vi "testIsTelQueueFull.vi"(8 "error in (no error)":errorcluster) -> (0 "error out":errorcluster)   [LabVIEW 2018]
doc: "Test the isTelQueueFull.vi."
uses:
  src/TcpServer/TcpServer.lvclass
  src/TcpServerTel/typedef/enqueueOptionsTypeDef.ctl
  src/TcpServerTel/typedef/queueOptionsTypeDef.ctl
  src/TcpServer/TcpServer.lvclass/TcpServer.ctl
  src/TcpServerTel/typedef/telTypeDef.ctl
  src/TcpServerBase/TcpServerBase.lvclass/TcpServerBase.ctl
  src/TcpServerTel/TcpServerTel.lvclass
  home/pcortes/github/ts_labview_tcp_json/src/TcpServerBase/TcpServerBase.lvclass
  <vilib>/addons/_JKI Toolkits/Caraya/classes/Assert/Assert False.vi
  <vilib>/addons/_JKI Toolkits/Caraya/classes/Assert/Assert True.vi
  <vilib>/addons/_JKI Toolkits/Caraya/classes/Test/Test.lvclass
  <vilib>/addons/_JKI Toolkits/Caraya/classes/Assert/Assert.lvclass
  src/TcpServerBase/TcpServerBase.lvclass
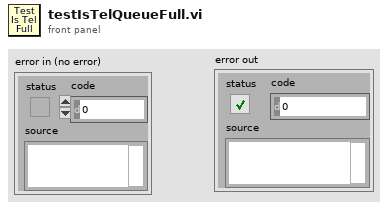
[diagram p1: front panel]
types:
  T1 = typedef "TcpServerTel.lvclass/enqueueOptionsTypeDef.ctl" = enum16{"lossy enqueue", "normal enqueue"}
  T2 = typedef "TcpServerTel.lvclass/queueOptionsTypeDef.ctl" = cluster{"EnqueueOptions":T1, "Timeout":i32}
  T3 = cluster{"cmdServerPort":u16, "telServerPort":u16, "serverTimeout (ms)":i32, "serverBytesToRead":i32, "telQueueServerMaxSize":i32, "EnqueueOptions":T1, "telQueueServerTimeout":i32, "tcpClientQueueMaxSize":i32}
  T4 = typedef "TcpServerTel.lvclass/telTypeDef.ctl" = cluster{"name":string, "telDetails":string}
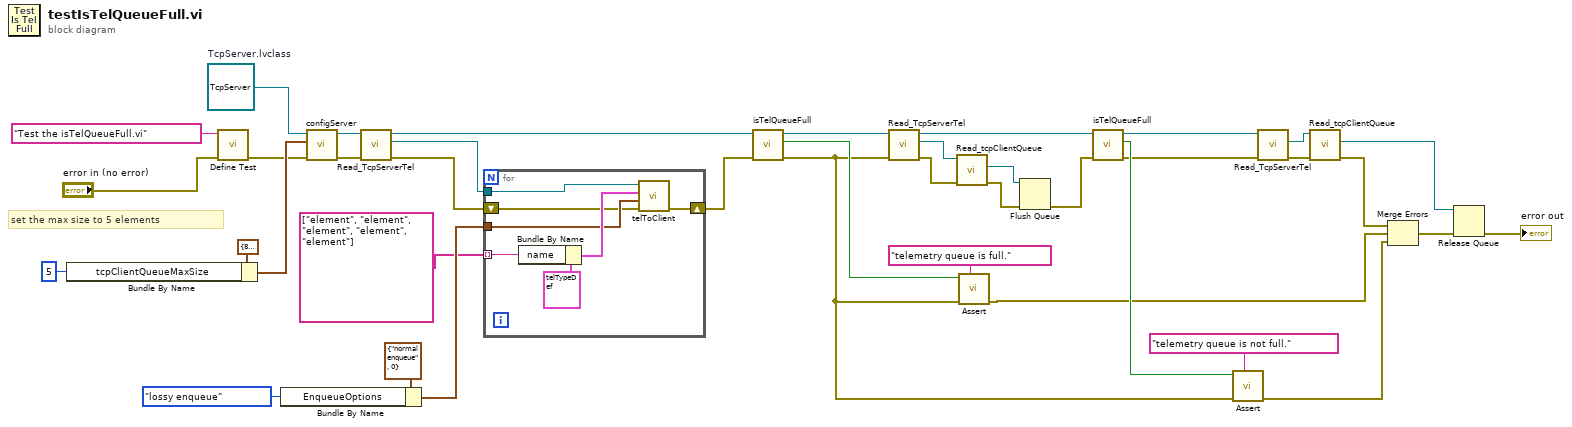
[diagram p0: block diagram]
diagram:
  w27 = refnum<class "TcpServer.lvclass"> refnum  # TcpServer.lvclass
  # "set the max size to 5 elements"
  n1 = Bundle By Name(cluster=T3 {"cmdServerPort"=8888, "telServerPort"=8888, "serverTimeout (ms)"=100, "serverBytesToRead"=32768, "telQueueServerMaxSize"=1000, "EnqueueOptions"=enum."lossy enqueue", "telQueueServerTimeout"=50, "tcpClientQueueMaxSize"=100} ("ServerConfiguration"), "tcpClientQueueMaxSize"=5 ("telQueueServerMaxSize")) -> (w26:T3)
  n2 = call <vilib>:"Define Test.vi"("error in (no error)"="error in (no error)", "Label (VI Title)"="Test the isTelQueueFull.vi") -> ("error out"=w25:errorcluster)  [unwired: 9 in]
  n3 = Bundle By Name(cluster=T2 {"EnqueueOptions"=enum."normal enqueue", "Timeout"=0} ("queueOptions"), "EnqueueOptions"=enqueueOptionsTypeDef."lossy enqueue") -> (w18:T2)
  n4 = call "configServer.vi"("error in (no error)"=w25, "ServerConfiguration"=w26, "tcpServer in"=w27) -> ("error out"=w23:errorcluster, "tcpServer out"=w24:refnum<class "TcpServer.lvclass">)  [unwired: 7 in]
  n5 = call "Read_TcpServerTel.vi"("error in (no error)"=w23, "TcpServer in"=w24) -> ("error out"=w21:errorcluster, "TcpServerTel.lvclass"=w22:refnum<class "TcpServerTel.lvclass">, "TcpServer out"=w17:refnum<class "TcpServer.lvclass">)  [unwired: 7 in]
  n6 = for {
    tunnel: w22 -> [w46]
    tunnel: w18 -> [w42]
    shift-right: [w40] -> w16
    shift-left: w21 -> [w41]
    tunnel: string[] ["element", "element", "element", "element", "element"] -> [w44] mode=indexing
    n7 = Bundle By Name(cluster=T4 {"name"="elevation", "telDetails"="\"compName\":\"MTMount\""} ("Telemetry"), "name"=w44) -> (w43:T4)
    n8 = call "telToClient.vi"("error in (no error)"=w41, "queueOptions"=w42, "Telemetry"=w43, "TcpServerTel in"=w46) -> ("error out"=w40:errorcluster)  [unwired: 6 in, 1 out]
  }
  n9 = call "isTelQueueFull.vi"("error in (no error)"=w16, "tcpServer in"=w17) -> ("error out"=w7:errorcluster, "isTelQueueFull"=w34:bool, "tcpServer out"=w13:refnum<class "TcpServer.lvclass">)  [unwired: 7 in]
  n10 = call "Read_TcpServerTel.vi"("error in (no error)"=w7, "TcpServer in"=w13) -> ("error out"=w14:errorcluster, "TcpServerTel.lvclass"=w15:refnum<class "TcpServerTel.lvclass">, "TcpServer out"=w10:refnum<class "TcpServer.lvclass">)  [unwired: 7 in]
  n11 = call "Read_tcpClientQueue.vi"("error in (no error)"=w14, "TcpServerBase in"=w15) -> ("error out"=w11:errorcluster, "tcpClientQueue"=w12:refnum<queue>)  [unwired: 7 in, 1 out]
  n12 = call-poly <vilib>:"Assert.vi"("Label"="telemetry queue is full.", "error in (no error)"=w7, "True?"=w34) -> ("error out"=w3:errorcluster)  [unwired: 8 in]
  n13 = Flush Queue(queue=w12, error in (no error)=w11) -> (error out=w9:errorcluster)  [unwired: 2 out]
  n14 = call "isTelQueueFull.vi"("error in (no error)"=w9, "tcpServer in"=w10) -> ("error out"=w4:errorcluster, "isTelQueueFull"=w6:bool, "tcpServer out"=w5:refnum<class "TcpServer.lvclass">)  [unwired: 7 in]
  n15 = call-poly <vilib>:"Assert.vi"("Label"="telemetry queue is not full.", "error in (no error)"=w7, "False?"=w6) -> ("error out"=w2:errorcluster)  [unwired: 8 in]
  n16 = call "Read_TcpServerTel.vi"("error in (no error)"=w4, "TcpServer in"=w5) -> ("error out"=w33:errorcluster, "TcpServerTel.lvclass"=w32:refnum<class "TcpServerTel.lvclass">)  [unwired: 7 in, 1 out]
  n17 = call "Read_tcpClientQueue.vi"("error in (no error)"=w33, "TcpServerBase in"=w32) -> ("error out"=w30:errorcluster, "tcpClientQueue"=w31:refnum<queue>)  [unwired: 7 in, 1 out]
  n18 = Merge Errors(w30, w3, w2) -> (w35:errorcluster)
  n19 = Release Queue(queue=w31, error in (no error)=w35) -> (error out=→"error out":errorcluster)  [unwired: 1 in, 2 out]
